vi "fgv_udp_lidar-data.vi"(7 "cmd":enum16{"init", "r-w", "read", "write", "close"}(ring), 8 "error in":errorcluster, 11 "data in":string) -> (0 "error out":errorcluster, 2 "recv_data":string, 3 "read":string)   [LabVIEW 2019]
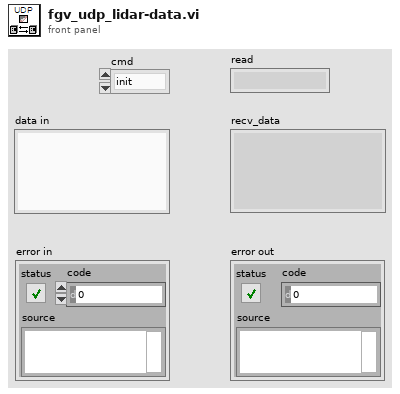
[diagram p1: front panel]
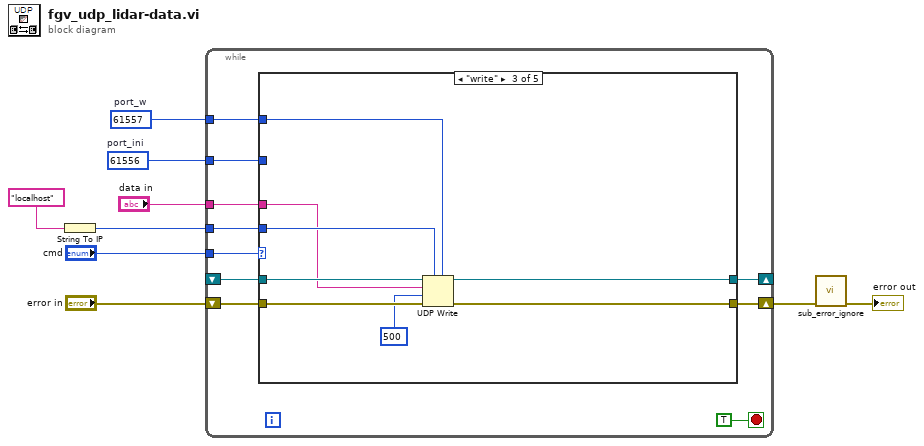
[diagram p0: block diagram]
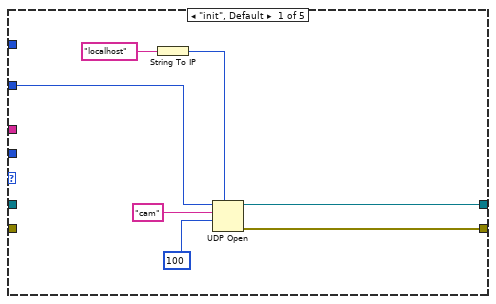
[diagram p2: hidden frame]
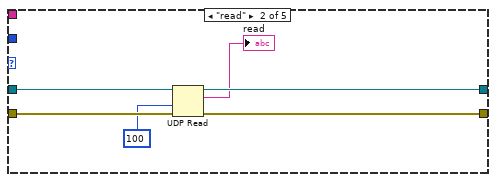
[diagram p3: hidden frame]
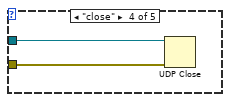
[diagram p4: hidden frame]
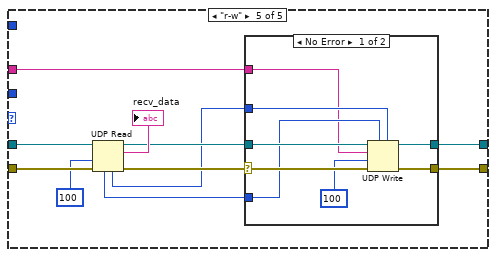
[diagram p5: hidden frame]
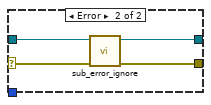
[diagram p6: hidden frame]
diagram:
  w1 = u16 61557  # port_w
  w2 = u16 61556  # port_ini
  n1 = String To IP(1:"localhost" ("Remote PC IP")) -> (0:w7:u32)
  n2 = while {
    tunnel: "cmd" -> [w18]
    shift-right: [w16] -> _
    shift-left: _ -> [w17]
    shift-right: [w15] -> w4
    shift-left: "error in" -> [w14]
    tunnel: w7 -> [w13]
    tunnel: "data in" -> [w12]
    tunnel: w2 -> [w11]
    tunnel: w1 -> [w10]
    stop <- TRUE stop-if-true
    n3 = case shown="\"write\"" w18 {
      tunnel: w17 -> [_ w32 w37 w42 w53]
      tunnel: [w26 w31 w38 _ w48] -> w16
      tunnel: [w25 w30 w39 _ w46] -> w15
      tunnel: w14 -> [_ w29 w40 w41 w51]
      tunnel: w13 -> [_ _ w36 _ _]
      tunnel: w12 -> [_ _ w35 _ w43]
      tunnel: w11 -> [w20 _ _ _ _]
      tunnel: w10 -> [_ _ w33 _ _]
      frame "init", Default {
        n4 = String To IP(1:"localhost") -> (0:w22:u32)
        n5 = UDP Open(7:w22, 9:100 ("타임아웃 ms (25000)"), 10:"cam" ("서비스 이름"), 11:w20) -> (port=w26:refnum<k16>, 0:w25:errorcluster)  [unwired: 1 in, 1 out]
      }
      frame "read" {
        n6 = UDP Read(connection ID=w32, timeout ms (25000)=100 ("타임아웃 ms (25000)"), 8:w29) -> (data out=→"read":string, error out=w30:errorcluster, 3:w31:refnum<k16>)  [unwired: 1 in, 2 out]
      }
      frame "write" {
        n7 = UDP Write(address=w36, port or service name=w33, connection ID=w37, data in=w35, 8:w40, 9:500 ("타임아웃 ms (25000)")) -> (error out=w39:errorcluster, 3:w38:refnum<k16>)
      }
      frame "close" {
        n8 = UDP Close(connection ID=w42, 8:w41) -> ()  [unwired: 2 out]
      }
      frame "r-w" {
        n9 = UDP Read(connection ID=w53, timeout ms (25000)=100, 8:w51) -> (data out=→"recv_data":string, error out=w49:errorcluster, 3:w47:refnum<k16>, 4:w44:u16, 6:w45:u32)  [unwired: 1 in]
        n10 = case shown="No Error" w49 {
          selector: w49 -> [w61 w63]
          tunnel: [w58 w64] -> w48
          tunnel: w47 -> [w60 w64]
          tunnel: [w59 w62] -> w46
          tunnel: w45 -> [w57 _]
          tunnel: w44 -> [w56 _]
          tunnel: w43 -> [w55 _]
          frame No Error {
            n11 = UDP Write(address=w57, port or service name=w56, connection ID=w60, data in=w55, 8:w61, 9:100 ("타임아웃 ms (25000)")) -> (error out=w59:errorcluster, 3:w58:refnum<k16>)
          }
          frame Error {
            n12 = call "sub_error_ignore.vi"("error in"=w63) -> ("error out"=w62:errorcluster)  [unwired: 10 in]
          }
        }
      }
    }
  }
  n13 = call "sub_error_ignore.vi"("error in"=w4) -> ("error out"=→"error out":errorcluster)  [unwired: 10 in]
